vi "capex write read global.vi"(6 "Bool in":bool[](array[boolean]), 7 "Value in":dbl[](array[numeric]), 8 "Channel":dbl=-1.0, 9 "Subsystem":T1(ring)=enum."relays", 10 "read/write":enum16{"read", "write"}(ring)=enum."write", 11 "Module":dbl) -> (0 "Single value":dbl, 1 "Single bool":bool, 2 "Value out":dbl[](array[numeric]), 4 "Bool out":bool[](array[boolean])=[TRUE, TRUE, FALSE, TRUE])   [LabVIEW 2013]
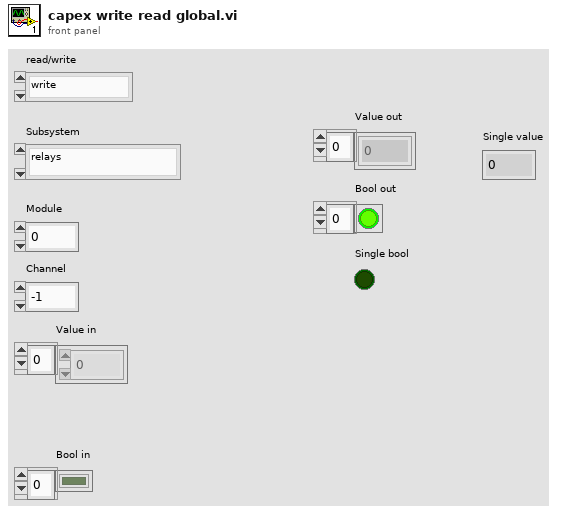
[diagram p1: front panel]
types:
  T1 = enum16{"GPIO", "chamber", "chiller", "analog out", "analog in", "DC power supply", "AC power supply", "thermocouples", "relays"}
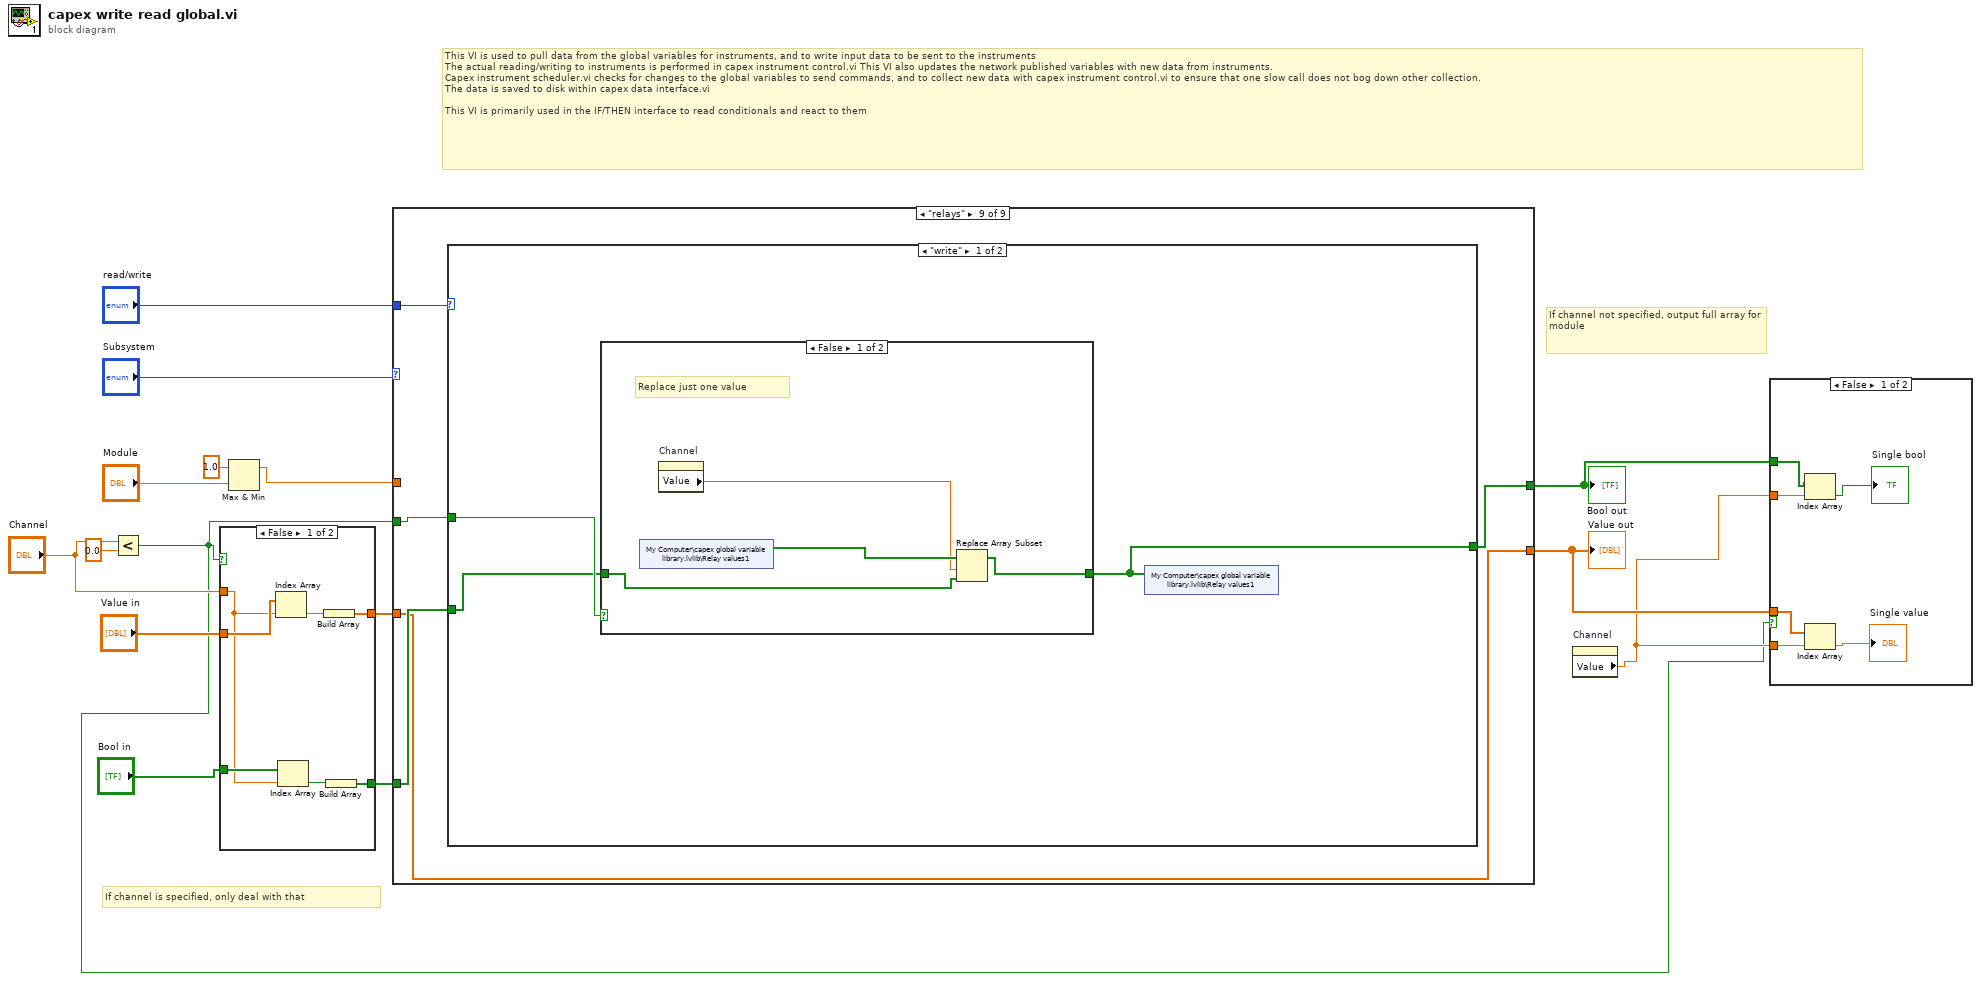
[diagram p0: block diagram]
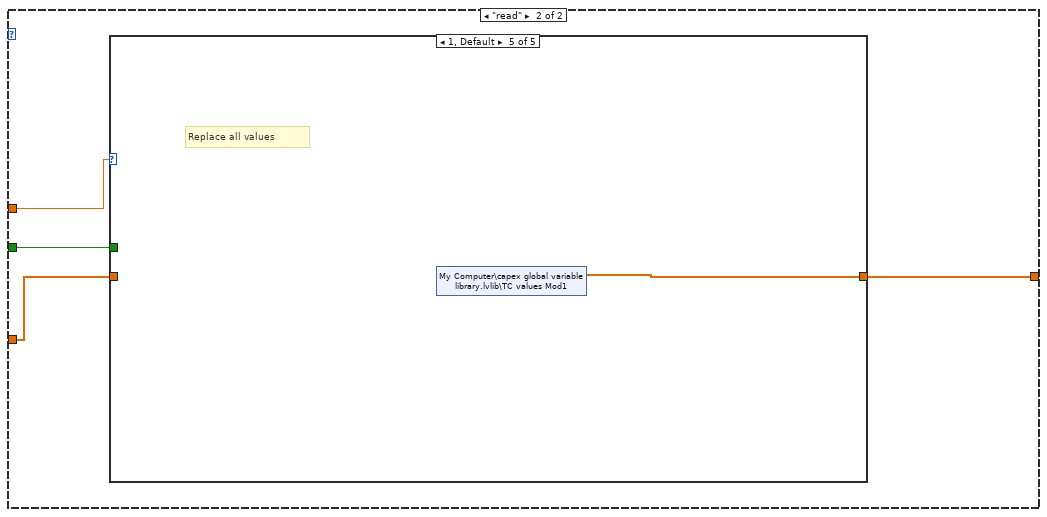
[diagram p5: hidden frame]
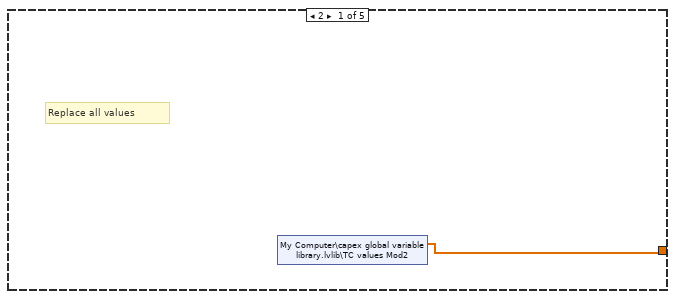
[diagram p6: hidden frame]
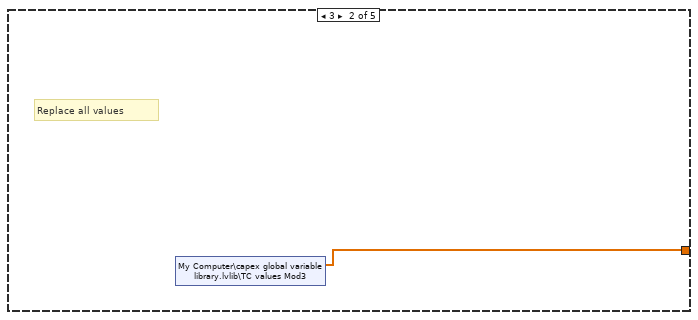
[diagram p7: hidden frame]
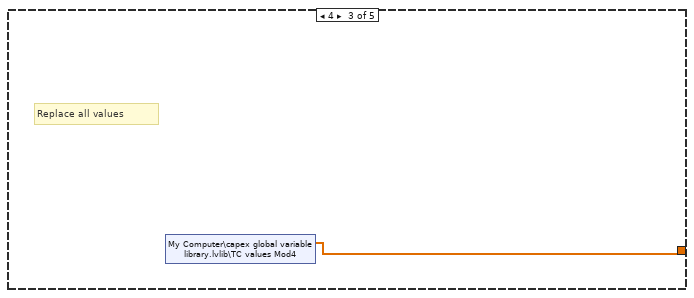
[diagram p8: hidden frame]
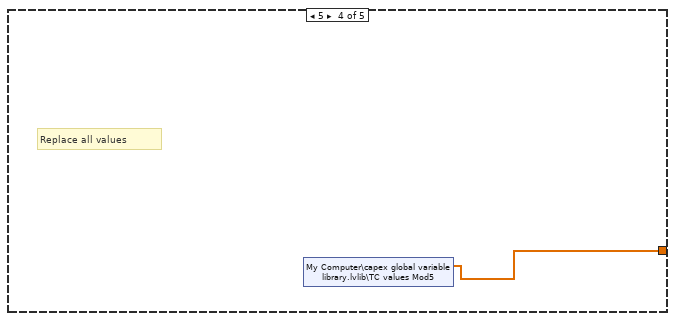
[diagram p9: hidden frame]
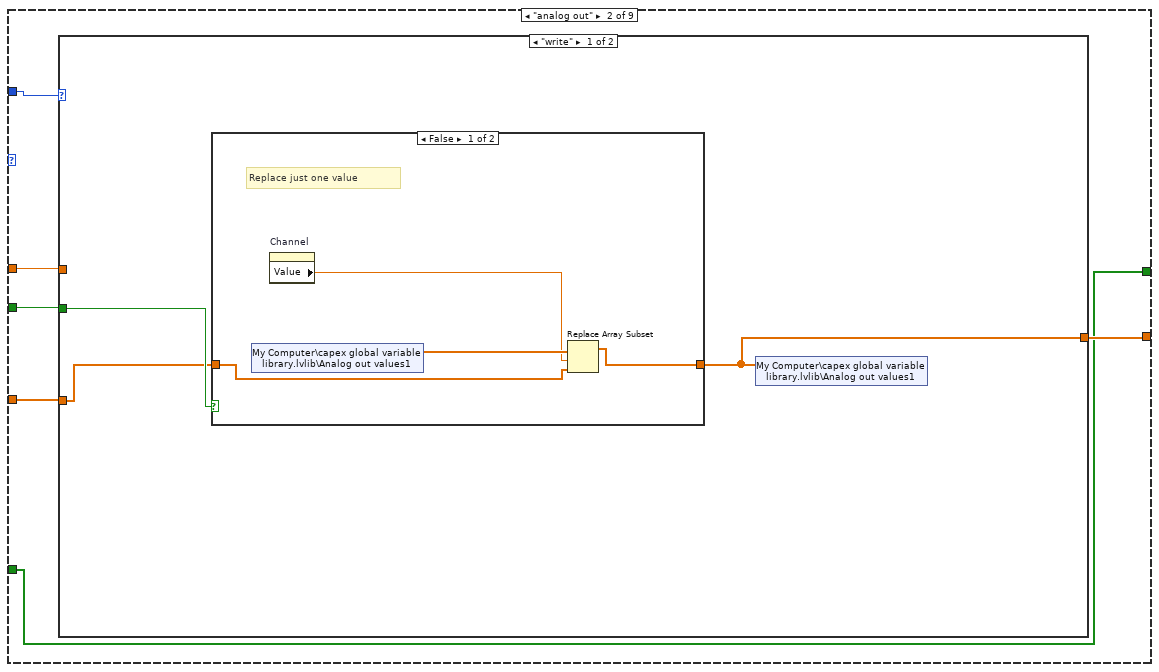
[diagram p10: hidden frame]
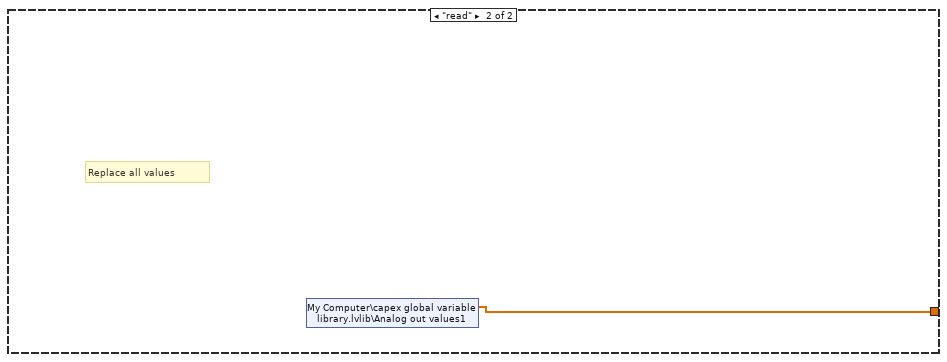
[diagram p12: hidden frame]
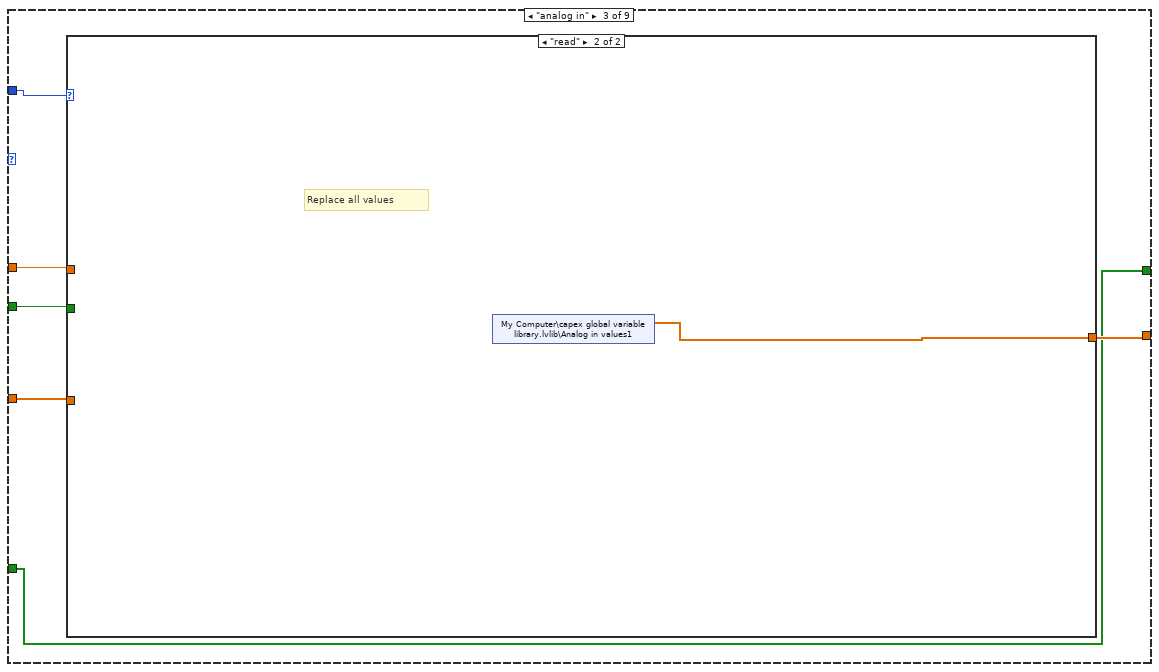
[diagram p13: hidden frame]
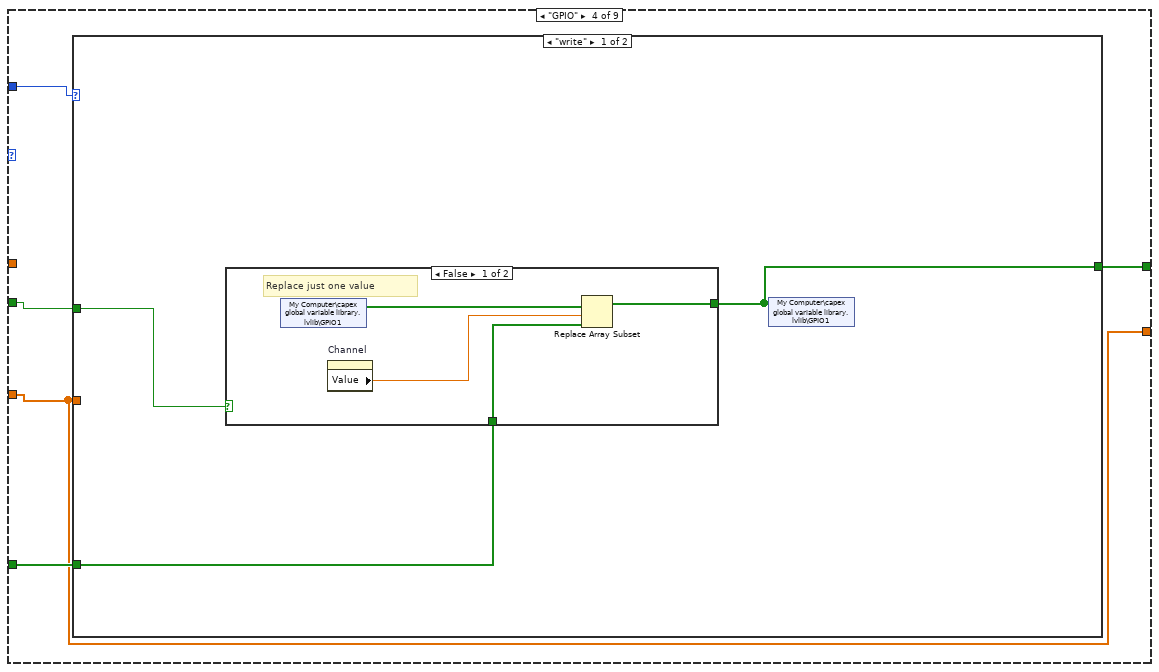
[diagram p15: hidden frame]
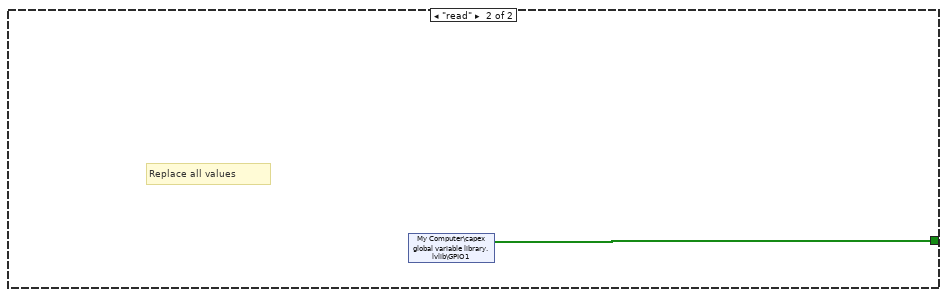
[diagram p17: hidden frame]
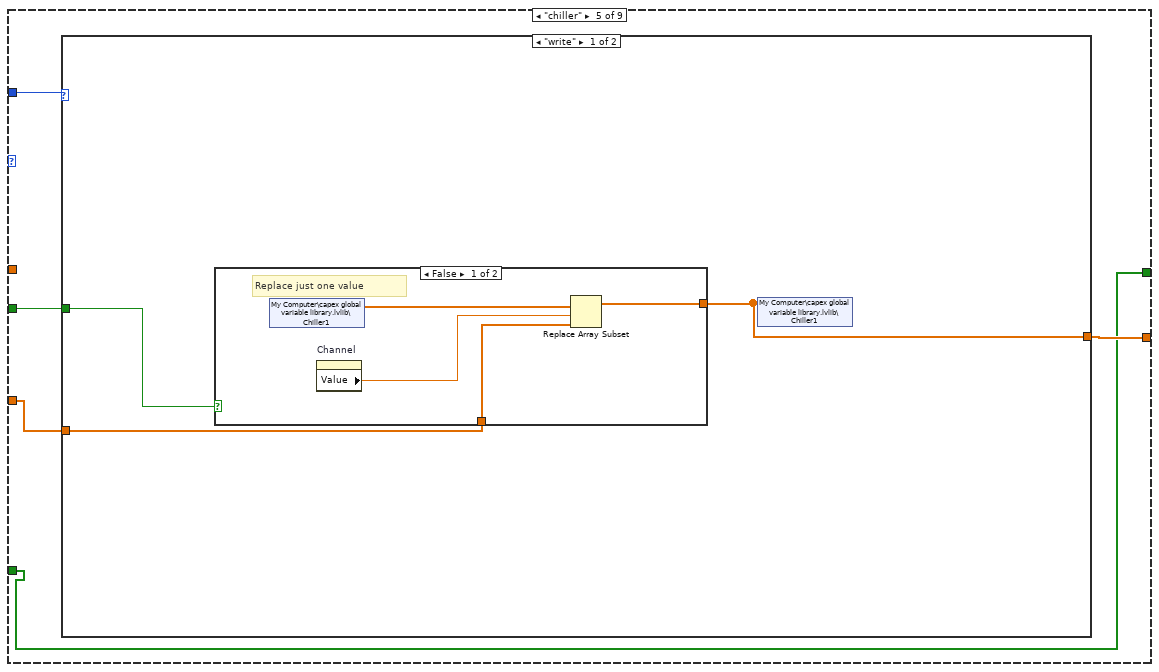
[diagram p18: hidden frame]
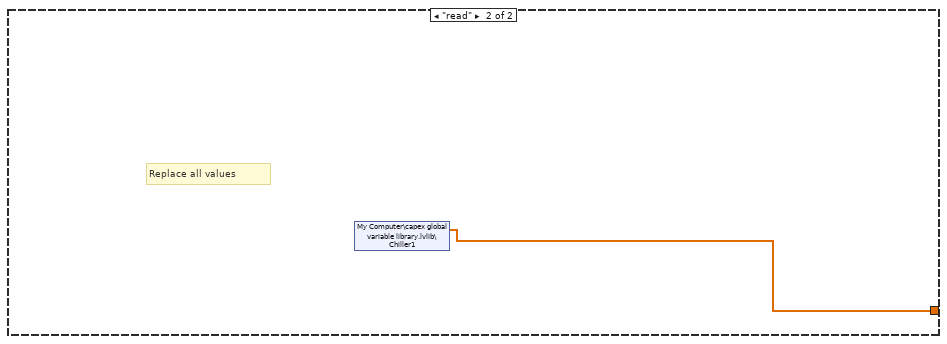
[diagram p20: hidden frame]
diagram:
  # "If channel is specified, only deal with that"
  # "This VI is used to pull data from the global variables for instruments, and to write input data to be sent to the instruments\nThe actual reading/writing to instruments is performed in capex instrument control.vi This VI also updates the network published variables with new data from instruments.\nCapex instrument scheduler.vi checks for changes to the global variables to send commands, and to collect new data with capex instrument control.vi to ensure that one slow call does not bog down other collection.\nThe data is saved to disk within capex data interface.vi\n\nThis VI is primarily used in the IF/THEN interface to read conditionals and react to them"
  # "If channel not specified, output full array for module"
  n1 = Less?(x="Channel", y=0.0) -> (x < y?=w2:bool)
  n2 = case shown="False" w2 {
    tunnel: "Value in" -> [w22 w24]
    tunnel: "Channel" -> [w18 _]
    tunnel: [w20 w24] -> w13
    tunnel: "Bool in" -> [w19 w23]
    tunnel: [w16 w23] -> w8
    frame False {
      n3 = Index Array(array=w22, index=w18) -> (element=w21:dbl)
      n4 = Index Array(array=w19, index=w18) -> (element=w17:bool)
      n5 = Build Array(w21) -> (w20:dbl[])
      n6 = Build Array(w17) -> (w16:bool[])
    }
    frame True {
    }
  }
  n7 = Max & Min(x=1.0, y="Module") -> (max(x,y)=w10:dbl)  [unwired: 1 out]
  n8 = case shown="\"relays\"" "Subsystem" {
    tunnel: "read/write" -> [w30 w46 w61 w64 w78 w93 w119 w150 w172]
    tunnel: w10 -> [w29 w45 w60 _ _ w92 w120 w154 _]
    tunnel: w13 -> [w28 w43 w58 w65 w81 w95 w123 w153 w174]
    tunnel: w2 -> [w27 w44 w59 w68 w82 w96 w124 w155 w173]
    tunnel: [w26 w42 w57 w65 w80 w94 w121 w151 w174] -> w12
    tunnel: [w25 w41 w56 w67 w79 w97 w122 w152 w176] -> w5
    tunnel: w8 -> [w25 w41 w56 w66 w79 w97 w122 w152 w175]
    frame "thermocouples" {
      n9 = case shown="\"write\"" w30 {
        tunnel: w29 -> [_ w35]
        tunnel: w28 -> [w31 w32]
        tunnel: w27 -> [_ w34]
        tunnel: [w31 w33] -> w26
        frame "write" {
        }
        frame "read" {
          n10 = case shown="1, Default" w35 {
            tunnel: w34 -> [_ _ _ _ _]
            tunnel: [w36 w37 w38 w39 w40] -> w33
            tunnel: w32 -> [_ _ _ _ _]
            frame 2 {
              # "Replace all values"
              n11 = shared-variable "My Computer\\capex global variable library.lvlib\\TC values Mod2"() -> (w36:dbl[])  [unwired: 1 in, 1 out]
            }
            frame 3 {
              # "Replace all values"
              n12 = shared-variable "My Computer\\capex global variable library.lvlib\\TC values Mod3"() -> (w37:dbl[])  [unwired: 1 in, 1 out]
            }
            frame 4 {
              # "Replace all values"
              n13 = shared-variable "My Computer\\capex global variable library.lvlib\\TC values Mod4"() -> (w38:dbl[])  [unwired: 1 in, 1 out]
            }
            frame 5 {
              # "Replace all values"
              n14 = shared-variable "My Computer\\capex global variable library.lvlib\\TC values Mod5"() -> (w39:dbl[])  [unwired: 1 in, 1 out]
            }
            frame 1, Default {
              # "Replace all values"
              n15 = shared-variable "My Computer\\capex global variable library.lvlib\\TC values Mod1"() -> (w40:dbl[])  [unwired: 1 in, 1 out]
            }
          }
        }
      }
    }
    frame "analog out" {
      n16 = case shown="\"write\"" w46 {
        tunnel: w45 -> [_ _]
        tunnel: w43 -> [w48 _]
        tunnel: w44 -> [w49 _]
        tunnel: [w47 w55] -> w42
        frame "write" {
          n17 = case shown="False" w49 {
            tunnel: [w53 w54] -> w47
            tunnel: w48 -> [w50 w54]
            frame False {
              # "Replace just one value"
              n18 = shared-variable "My Computer\\capex global variable library.lvlib\\Analog out values1"() -> (w52:dbl[])  [unwired: 1 in, 1 out]
              n19 = property on="Channel" class="DigNum (strict)"() -> ("Value"=w51:dbl)  [unwired: 2 in, 2 out]
              n20 = Replace Array Subset(array=w52, new element=w50, index=w51) -> (w53:dbl[])
            }
            frame True {
              # "Replace all values"
            }
          }
          n21 = shared-variable "My Computer\\capex global variable library.lvlib\\Analog out values1"(w47) -> ()  [unwired: 1 in, 1 out]
        }
        frame "read" {
          # "Replace all values"
          n22 = shared-variable "My Computer\\capex global variable library.lvlib\\Analog out values1"() -> (w55:dbl[])  [unwired: 1 in, 1 out]
        }
      }
    }
    frame "analog in" {
      n23 = case shown="\"read\"" w61 {
        tunnel: w60 -> [_ _]
        tunnel: w58 -> [w62 _]
        tunnel: w59 -> [_ _]
        tunnel: [w62 w63] -> w57
        frame "write" {
        }
        frame "read" {
          # "Replace all values"
          n24 = shared-variable "My Computer\\capex global variable library.lvlib\\Analog in values1"() -> (w63:dbl[])  [unwired: 1 in, 1 out]
        }
      }
    }
    frame "GPIO" {
      n25 = case shown="\"write\"" w64 {
        tunnel: w65 -> [_ _]
        tunnel: w68 -> [w71 _]
        tunnel: [w69 w77] -> w67
        tunnel: w66 -> [w70 _]
        frame "write" {
          n26 = case shown="False" w71 {
            tunnel: w70 -> [w74 w76]
            tunnel: [w72 w76] -> w69
            frame False {
              # "Replace just one value"
              n27 = shared-variable "My Computer\\capex global variable library.lvlib\\GPIO1"() -> (w73:bool[])  [unwired: 1 in, 1 out]
              n28 = property on="Channel" class="DigNum (strict)"() -> ("Value"=w75:dbl)  [unwired: 2 in, 2 out]
              n29 = Replace Array Subset(array=w73, new element=w74, index=w75) -> (w72:bool[])
            }
            frame True {
              # "Replace all values"
            }
          }
          n30 = shared-variable "My Computer\\capex global variable library.lvlib\\GPIO1"(w69) -> ()  [unwired: 1 in, 1 out]
        }
        frame "read" {
          # "Replace all values"
          n31 = shared-variable "My Computer\\capex global variable library.lvlib\\GPIO1"() -> (w77:bool[])  [unwired: 1 in, 1 out]
        }
      }
    }
    frame "chiller" {
      n32 = case shown="\"write\"" w78 {
        tunnel: w82 -> [w85 _]
        tunnel: [w84 w91] -> w80
        tunnel: w81 -> [w83 _]
        frame "write" {
          n33 = case shown="False" w85 {
            tunnel: w83 -> [w88 w90]
            tunnel: [w86 w90] -> w84
            frame False {
              # "Replace just one value"
              n34 = shared-variable "My Computer\\capex global variable library.lvlib\\Chiller1"() -> (w87:dbl[])  [unwired: 1 in, 1 out]
              n35 = property on="Channel" class="DigNum (strict)"() -> ("Value"=w89:dbl)  [unwired: 2 in, 2 out]
              n36 = Replace Array Subset(array=w87, new element=w88, index=w89) -> (w86:dbl[])
            }
            frame True {
              # "Replace all values"
            }
          }
          n37 = shared-variable "My Computer\\capex global variable library.lvlib\\Chiller1"(w84) -> ()  [unwired: 1 in, 1 out]
        }
        frame "read" {
          # "Replace all values"
          n38 = shared-variable "My Computer\\capex global variable library.lvlib\\Chiller1"() -> (w91:dbl[])  [unwired: 1 in, 1 out]
        }
      }
    }
    frame "chamber" {
      n39 = case shown="\"write\"" w93 {
        tunnel: w96 -> [w101 _]
        tunnel: [w100 w118] -> w94
        tunnel: w95 -> [w99 _]
        tunnel: w92 -> [w98 _]
        frame "write" {
          n40 = case shown="2" w98 {
            tunnel: w101 -> [w102 w112]
            tunnel: [w104 w111] -> w100
            tunnel: w99 -> [w103 w110]
            frame 1, Default {
              n41 = case shown="False" w102 {
                tunnel: w103 -> [w107 w109]
                tunnel: [w105 w109] -> w104
                frame False {
                  # "Replace just one value"
                  n42 = shared-variable "My Computer\\capex global variable library.lvlib\\Little chamber values1"() -> (w106:dbl[])  [unwired: 1 in, 1 out]
                  n43 = property on="Channel" class="DigNum (strict)"() -> ("Value"=w108:dbl)  [unwired: 2 in, 2 out]
                  n44 = Replace Array Subset(array=w106, new element=w107, index=w108) -> (w105:dbl[])
                }
                frame True {
                  # "Replace all values"
                }
              }
              n45 = shared-variable "My Computer\\capex global variable library.lvlib\\Little chamber values1"(w104) -> ()  [unwired: 1 in, 1 out]
            }
            frame 2 {
              n46 = case shown="False" w112 {
                tunnel: w110 -> [w115 w117]
                tunnel: [w113 w117] -> w111
                frame False {
                  # "Replace just one value"
                  n47 = shared-variable "My Computer\\capex global variable library.lvlib\\Big chamber values1"() -> (w114:dbl[])  [unwired: 1 in, 1 out]
                  n48 = property on="Channel" class="DigNum (strict)"() -> ("Value"=w116:dbl)  [unwired: 2 in, 2 out]
                  n49 = Replace Array Subset(array=w114, new element=w115, index=w116) -> (w113:dbl[])
                }
                frame True {
                  # "Replace all values"
                }
              }
              n50 = shared-variable "My Computer\\capex global variable library.lvlib\\Big chamber values1"(w111) -> ()  [unwired: 1 in, 1 out]
            }
          }
        }
        frame "read" {
          # "Replace all values"
          n51 = shared-variable "My Computer\\capex global variable library.lvlib\\Big chamber values1"() -> (w118:dbl[])  [unwired: 1 in, 1 out]
        }
      }
    }
    frame "AC power supply" {
      n52 = case shown="\"write\"" w119 {
        tunnel: w123 -> [w127 _]
        tunnel: w124 -> [w128 w147]
        tunnel: [w126 w146] -> w121
        tunnel: w120 -> [w125 w145]
        frame "write" {
          n53 = case shown="1, Default" w125 {
            tunnel: w128 -> [w131 w138]
            tunnel: w127 -> [w130 w139]
            tunnel: [w129 w137] -> w126
            frame 1, Default {
              n54 = case shown="False" w131 {
                tunnel: [w134 w136] -> w129
                tunnel: w130 -> [w132 w136]
                frame False {
                  # "Replace just one value"
                  n55 = shared-variable "My Computer\\capex global variable library.lvlib\\AC power supply1"() -> (w135:dbl[])  [unwired: 1 in, 1 out]
                  n56 = property on="Channel" class="DigNum (strict)"() -> ("Value"=w133:dbl)  [unwired: 2 in, 2 out]
                  n57 = Replace Array Subset(array=w135, new element=w132, index=w133) -> (w134:dbl[])
                }
                frame True {
                  # "Replace all values"
                }
              }
              n58 = shared-variable "My Computer\\capex global variable library.lvlib\\AC power supply1"(w129) -> ()  [unwired: 1 in, 1 out]
            }
            frame 2 {
              n59 = case shown="False" w138 {
                tunnel: [w142 w144] -> w137
                tunnel: w139 -> [w140 w144]
                frame False {
                  # "Replace just one value"
                  n60 = shared-variable "My Computer\\capex global variable library.lvlib\\AC power supply1"() -> (w143:dbl[])  [unwired: 1 in, 1 out]
                  n61 = property on="Channel" class="DigNum (strict)"() -> ("Value"=w141:dbl)  [unwired: 2 in, 2 out]
                  n62 = Replace Array Subset(array=w143, new element=w140, index=w141) -> (w142:dbl[])
                }
                frame True {
                  # "Replace all values"
                }
              }
              n63 = shared-variable "My Computer\\capex global variable library.lvlib\\AC power supply1"(w137) -> ()  [unwired: 1 in, 1 out]
            }
          }
        }
        frame "read" {
          n64 = case shown="1, Default" w145 {
            tunnel: w147 -> [_ _]
            tunnel: [w148 w149] -> w146
            frame 2 {
              # "Replace all values"
              n65 = shared-variable "My Computer\\capex global variable library.lvlib\\AC power supply2"() -> (w148:dbl[])  [unwired: 1 in, 1 out]
            }
            frame 1, Default {
              # "Replace all values"
              n66 = shared-variable "My Computer\\capex global variable library.lvlib\\AC power supply1"() -> (w149:dbl[])  [unwired: 1 in, 1 out]
            }
          }
        }
      }
    }
    frame "DC power supply" {
      n67 = case shown="\"write\"" w150 {
        tunnel: w153 -> [w158 _]
        tunnel: w155 -> [w159 w170]
        tunnel: [w157 w169] -> w151
        tunnel: w154 -> [w156 w168]
        frame "write" {
          n68 = case shown="1, Default" w156 {
            tunnel: w159 -> [w162]
            tunnel: w158 -> [w161]
            tunnel: [w160] -> w157
            frame 1, Default {
              n69 = case shown="False" w162 {
                tunnel: [w165 w167] -> w160
                tunnel: w161 -> [w163 w167]
                frame False {
                  # "Replace just one value"
                  n70 = shared-variable "My Computer\\capex global variable library.lvlib\\DC power supply1"() -> (w166:dbl[])  [unwired: 1 in, 1 out]
                  n71 = property on="Channel" class="DigNum (strict)"() -> ("Value"=w164:dbl)  [unwired: 2 in, 2 out]
                  n72 = Replace Array Subset(array=w166, new element=w163, index=w164) -> (w165:dbl[])
                }
                frame True {
                  # "Replace all values"
                }
              }
              n73 = shared-variable "My Computer\\capex global variable library.lvlib\\DC power supply1"(w160) -> ()  [unwired: 1 in, 1 out]
            }
          }
        }
        frame "read" {
          n74 = case shown="1, Default" w168 {
            tunnel: w170 -> [_]
            tunnel: [w171] -> w169
            frame 1, Default {
              # "Replace all values"
              n75 = shared-variable "My Computer\\capex global variable library.lvlib\\DC power supply1"() -> (w171:dbl[])  [unwired: 1 in, 1 out]
            }
          }
        }
      }
    }
    frame "relays" {
      n76 = case shown="\"write\"" w172 {
        tunnel: w175 -> [w178 _]
        tunnel: w173 -> [w179 _]
        tunnel: [w177 w185] -> w176
        frame "write" {
          n77 = case shown="False" w179 {
            tunnel: [w183 w184] -> w177
            tunnel: w178 -> [w180 w184]
            frame False {
              # "Replace just one value"
              n78 = shared-variable "My Computer\\capex global variable library.lvlib\\Relay values1"() -> (w182:bool[])  [unwired: 1 in, 1 out]
              n79 = property on="Channel" class="DigNum (strict)"() -> ("Value"=w181:dbl)  [unwired: 2 in, 2 out]
              n80 = Replace Array Subset(array=w182, new element=w180, index=w181) -> (w183:bool[])
            }
            frame True {
              # "Replace all values"
            }
          }
          n81 = shared-variable "My Computer\\capex global variable library.lvlib\\Relay values1"(w177) -> ()  [unwired: 1 in, 1 out]
        }
        frame "read" {
          # "Replace all values"
          n82 = shared-variable "My Computer\\capex global variable library.lvlib\\Relay values1"() -> (w185:bool[])  [unwired: 1 in, 1 out]
        }
      }
    }
  }
  "Value out" <- w12
  "Bool out" <- w5
  n83 = property on="Channel" class="DigNum (strict)"() -> ("Value"=w6:dbl)  [unwired: 2 in, 2 out]
  n84 = case shown="False" w2 {
    tunnel: w12 -> [w191 _]
    tunnel: w6 -> [w190 _]
    tunnel: w6 -> [w187 _]
    tunnel: w5 -> [w186 _]
    frame False {
      n85 = Index Array(array=w186, index=w187) -> (element=→"Single bool":bool)
      n86 = Index Array(array=w191, index=w190) -> (element=→"Single value":dbl)
    }
    frame True {
    }
  }
